vi "4309 multi test with switch.vi"() -> ()   [LabVIEW 2019]
uses:
  Chart_Graph_Mean_Range_StdDev.ctl
  <vilib>/Analysis/baseanly.llb/Mean (DBL).vi
  <vilib>/Analysis/NI_AALBase.lvlib
panel:
  in  "DMM 7.5 Digits All 4 Channels":dbl[][](array[numeric])=[[3.4835981189908805, 3.4835973578772146, 3.4835977893402292, 3.483597533766503, 3.4835975009361055, 3.4835974259988975, 3.4835978392404665, 3.483597710153336, 3.483597530409142, 3.483597982965577, 3.4835974835927273, 3.4835975661067864, 3.4835978929675346, 3.483597859704548, 3.483597570043803, 3.48359758877419, 3.483597718635417, 3.4835974386993853, 3.4835979909144443, 3.483597546796911, 3.483597791629489, 3.4835976928422, 3.4835977006392365, 3.4835976984527726, 3.4835973562416775, 3.483597995505588, 3.483597815535534, 3.4835978300326116, 3.483597985892642, 3.483597413809255, 3.483597723962119, 3.4835979022635915, 3.4835977166666647, 3.483597588468151, 3.483598009044623, 3.4835974566412133, 3.4835975839370192, 3.4835975376641026, 3.483597439503911, 3.483597317956866, 3.4835972485909776, 3.4835976458862903, 3.4835976825108617, 3.48359823081158, 3.4835976718930137, 3.4835976585808193, 3.4835978362135966, 3.483597507818025, 3.483597799164003, 3.483597349716458, 3.4835975948182454, 3.4835981329699433, 3.4835979467910407, 3.4835974912342884, 3.4835974532960456, 3.483597903200004, 3.483597374049583, 3.483597334623242, 3.483597710860957, 3.483597692009984, 3.4835976586327315, 3.4835977598936534, 3.4835979763023603, 3.4835975896116587, 3.4835978971434263, 3.4835976281822316, 3.4835982271082013, 3.4835976949272403, 3.4835974320575938, 3.483597408013519, 3.4835976534048685, 3.48359766337321, 3.483597430968089, 3.4835978228589006, 3.4835977691488273, 3.4835979109499484, 3.483597518460395, 3.483597806961959, 3.483597578691926, 3.4835975527599476, 3.483597860450459, 3.4835974511972227, 3.4835973978219275, 3.4835975280386107, 3.4835970961662297, 3.4835979186960975, 3.483597285920934, 3.483597386907896, 3.483597474535041, 3.4835973080741587, 3.4835975196582534, 3.4835974480673357, 3.4835976798422204, 3.483597547235268, 3.483597484346667, 3.483597539878841, 3.483597791092996, 3.483597598658644, 3.48359767066429, 3.4835976010356733, 3.4835977898228307, 3.483597544054286, 3.4835971331899516, 3.4835975044953993, 3.4835974626533996, 3.483597132727585, 3.4835975524889027, 3.4835979535117207, 3.4835972493429948, 3.483597640255253, 3.4835974086907697, 3.4835973506672318, 3.483597580088908, 3.483597239500539, 3.483597486011177, 3.4835975002194246, 3.483597090891085, 3.483597714859873, 3.4835976666442754, 3.4835972680152745, 3.4835977448807194, 3.483597350763673, 3.4835973529914943, 3.4835976118884404, 3.4835975154265597, 3.483597695000821, 3.4835974558961684, 3.483597790103636], [3.4850700897521563, 3.485070233425622, 3.4850703496943347, 3.4850708481529473, 3.485070572181595, 3.485070105960937, 3.485070465485683, 3.4850704480083396, 3.48507056459965, 3.4850708183835595, 3.4850708166846527, 3.485070796405387, 3.4850707761851427, 3.485070608667662, 3.4850707882696508, 3.4850707241151975, 3.4850706596362566, 3.48507073021978, 3.485070567481813, 3.4850707162760663, 3.485070893790592, 3.4850704393547267, 3.485070651192876, 3.485070267833332, 3.4850708914554103, 3.4850705970227684, 3.4850705496821712, 3.485070893808849, 3.485070908236491, 3.4850704723673553, 3.4850706194869305, 3.4850704541132527, 3.4850707021341325, 3.4850710097049173, 3.4850709609995607, 3.4850706992583946, 3.4850710502732944, 3.4850708242361663, 3.485071009568022, 3.4850706205187802, 3.4850704634402474, 3.4850708131553314, 3.485070283346761, 3.485070802639425, 3.4850707294320875, 3.4850710718142284, 3.48507067385808, 3.4850708139996227, 3.4850706485313316, 3.485071205234073, 3.4850708802082133, 3.485070539592214, 3.4850703284695643, 3.485070644610402, 3.4850706377352365, 3.485070724333666, 3.485070706865352, 3.485071039978291, 3.4850708932740937, 3.4850703374231804, 3.4850706519379795, 3.4850704993977777, 3.4850704497575355, 3.4850705472916865, 3.4850708830277983, 3.4850702392811503, 3.48507065435932, 3.4850707605356352, 3.4850706390730855, 3.4850704744759575, 3.4850708749760537, 3.4850704959682712, 3.48507057686368, 3.485070482100544, 3.485070110520969, 3.4850708314094643, 3.4850704513493116, 3.485070655338042, 3.4850698942787095, 3.485070641499467, 3.485070060001174, 3.485070454200556, 3.485070688596838, 3.4850706243046936, 3.485070579152903, 3.485069883099495, 3.485070062034084, 3.485070525913557, 3.485070210088132, 3.485070026034661, 3.4850702456185907, 3.485070243940185, 3.4850697001719446, 3.4850702521018917, 3.4850700772887624, 3.4850700859590287, 3.485070371774776, 3.4850700961734526, 3.485070172855618, 3.485069905757029, 3.4850703159307965, 3.4850698537426226, 3.485070462070553, 3.4850699512833727, 3.4850698464028094, 3.4850699259717026, 3.4850701371431896, 3.4850702401475635, 3.485070006300969, 3.485070088453557, 3.4850701595221656, 3.485070253223072, 3.4850696208469243, 3.4850698353777982, 3.48506973491397, 3.4850699043293396, 3.485069909154778, 3.485069945468628, 3.4850700162729797, 3.4850700637961176, 3.4850698568711835, 3.485069683841688, 3.485069930522382, 3.48506970179727, 3.485070116146578, 3.485070421850128, 3.485070158963441, 3.4850698427039397], [3.481571899555477, 3.4815720996809536, 3.481572168540679, 3.481572401004205, 3.4815723090577384, 3.481571988546094, 3.4815728274152624, 3.4815728062014335, 3.481572501577856, 3.481572607429995, 3.481572610595567, 3.4815725639158046, 3.4815731629523547, 3.48157245445838, 3.481572678822192, 3.481572529789867, 3.4815725819006804, 3.481572967069484, 3.4815731074475686, 3.481572693006066, 3.4815728208347263, 3.481572524099559, 3.481573131123811, 3.4815725324422293, 3.4815725721654815, 3.4815727955137086, 3.4815732409351097, 3.48157252834275, 3.481572511998337, 3.4815730302590793, 3.481572830362119, 3.4815731395241, 3.48157304282813, 3.481573010928663, 3.4815726753855367, 3.481573126747513, 3.4815728716190883, 3.481572781318836, 3.481572732683734, 3.4815727357820037, 3.481572704616765, 3.481572784355119, 3.4815728763523865, 3.4815728056849347, 3.481572474565925, 3.4815728651620326, 3.481572960730617, 3.4815730411537085, 3.4815726474348017, 3.4815728656925575, 3.4815728037625746, 3.4815725683714147, 3.4815727765135653, 3.481572602782018, 3.4815725196736356, 3.4815723014267093, 3.481572220656706, 3.481572534362172, 3.4815728413086053, 3.481572371815714, 3.481572564065832, 3.4815724851708483, 3.4815726220738314, 3.481572401586816, 3.481572213900522, 3.481572531080011, 3.4815726736061214, 3.481572174946321, 3.4815728025844557, 3.481572249370352, 3.4815721671205733, 3.481572565457693, 3.481572360373885, 3.4815726824797832, 3.481572841781139, 3.481572643049169, 3.4815721595516465, 3.4815723952810407, 3.481572162387346, 3.4815727239032985, 3.4815723917459103, 3.4815720794809555, 3.4815722693538627, 3.4815725743888026, 3.4815720485747352, 3.481572470689445, 3.4815725915569478, 3.4815727324723182, 3.4815724521032285, 3.4815727954319797, 3.4815721995573847, 3.4815721839029323, 3.4815721980816043, 3.4815721160737434, 3.481572277861212, 3.4815721507038226, 3.481572288856155, 3.481572226063303, 3.4815719656002706, 3.481572592875911, 3.481572194406493, 3.481572412416302, 3.481572084967407, 3.4815721696802724, 3.4815720226137596, 3.48157205650772, 3.48157190538414, 3.481572045063342, 3.481572018317761, 3.481572185489624, 3.481572154901699, 3.481571926660422, 3.4815718999626237, 3.4815721280737373, 3.481572224094029, 3.481572353081591, 3.481572261017972, 3.481571975995548, 3.481572128201471, 3.481572180067718, 3.4815715655143373, 3.4815718214629943, 3.4815715789142585, 3.4815719255662994, 3.4815718246399183, 3.481571977351035, 3.481571843104722, 3.4815719523213], [3.484305724115568, 3.4843058305875227, 3.4843062901111512, 3.484305936231965, 3.4843057288438772, 3.4843064559020687, 3.4843063293991383, 3.4843062952127486, 3.4843066955825175, 3.484306829330163, 3.4843061981418333, 3.4843063620415697, 3.484306236532934, 3.4843064437456763, 3.4843061743985606, 3.484306186782022, 3.484306270580653, 3.484306740665737, 3.4843061208250283, 3.484305965882024, 3.484306590076414, 3.4843059649148156, 3.4843062673844587, 3.4843060655731373, 3.484306302924423, 3.484306432337808, 3.484306632080742, 3.484306009373001, 3.484306543172826, 3.484306382441485, 3.4843062427876945, 3.4843061764316796, 3.48430660308128, 3.4843062004511594, 3.4843060610943404, 3.4843068333436076, 3.484306621812408, 3.484306649840404, 3.484306285295565, 3.4843059813072683, 3.484306553789793, 3.4843062824735846, 3.484306430756184, 3.4843068757434295, 3.484306442887929, 3.4843065762633945, 3.484305988738697, 3.4843066243270724, 3.484306445500346, 3.484306832441937, 3.4843060150056067, 3.4843063781220796, 3.4843066789757673, 3.4843064150739504, 3.4843061381565823, 3.484305675942912, 3.4843062793645334, 3.4843063841371547, 3.484306272484438, 3.4843062706304226, 3.484306376440192, 3.484305708893772, 3.484306251000281, 3.484306233665289, 3.4843063068999873, 3.4843062524955, 3.4843063590903363, 3.484305999586689, 3.4843062500567994, 3.4843060777149777, 3.484305966811333, 3.4843060316739654, 3.4843057546627394, 3.484306023228924, 3.4843061239924005, 3.4843060196427316, 3.4843055330739823, 3.4843056881987136, 3.484305713110319, 3.484306038013802, 3.484305910294656, 3.4843055487391927, 3.484305955637334, 3.4843058755725593, 3.4843058736827315, 3.4843058395981483, 3.4843057942888587, 3.4843056863141157, 3.484305964223715, 3.4843061658501737, 3.4843061897594634, 3.484305738279498, 3.484305518799016, 3.484305825857164, 3.484306035291972, 3.484306102538148, 3.484305819322618, 3.4843057482448683, 3.4843055381532038, 3.484305561533999, 3.48430561697876, 3.484305709331289, 3.484305709513193, 3.4843057764415675, 3.484305845716869, 3.4843058548617227, 3.4843058558332802, 3.4843060036480638, 3.484306017456, 3.4843051117756003, 3.4843054695551543, 3.484305914306639, 3.4843058242771217, 3.4843058614305953, 3.4843052097363807, 3.4843056026459474, 3.484305395133235, 3.4843055297155088, 3.484305541519446, 3.4843059349268186, 3.4843053694848685, 3.4843057348549347, 3.484305160045847, 3.484304944580094, 3.4843056614719075, 3.4843052011624254, 3.4843052966632158, 3.484305352531343]]
  in  "Take New DMM 7.5 Digit Measurements":bool
  out "error values of channels":dbl[][](array[numeric])=[[3.916877821419362e-05, 3.708869139362747e-06, 3.813682889530767e-05, 5.939885534989031e-06], [3.635893304743121e-05, -1.4762659956701896e-06, 3.541455057165521e-05, 6.165901756727266e-06], [3.8312583618971274e-05, 5.44234072030747e-07, 3.851021763967566e-05, 6.687408843131237e-06], [3.683071982907293e-05, 6.149038647151883e-07, 3.84443079650687e-05, 7.168960555414827e-06], [3.3856852708513685e-05, -2.440297388606183e-06, 3.5546966388633194e-05, 6.810853058869526e-06], [3.645943377117433e-05, 4.1571643194515673e-07, 3.861609064648164e-05, 7.510668457832992e-06], [3.376470219373928e-05, -2.523192756953563e-06, 3.560124494406125e-05, 7.423303348019772e-06], [3.310682505075491e-05, -1.8358768398840652e-06, 3.552758119029775e-05, 7.75010252906938e-06], [3.651997278319996e-05, 1.7017873870095457e-06, 3.969301297601646e-05, 8.367025434719011e-06], [3.8678501685485145e-05, 2.61423281289197e-06, 4.1762457464233904e-05, 1.1427786008599838e-05], [4.814853281098763e-05, 1.5347319277658755e-05, 4.9363542874658606e-05, 1.8916138766034152e-05], [5.463157506069294e-05, 2.148276930480364e-05, 5.719963653616489e-05, 3.198721146668859e-05]] format="%#_6p"
  out "Results Output":T1={"ch3 range"=1.4045208578838952e-05, "ch3 std dev"=3.830360581374409e-06, "ch3 mean"=3.484274052845448, "Histogram Graph ch3"={"X Values"=[3.484267646031002, 3.48426905055186, 3.4842704550727177, 3.4842718595935755, 3.4842732641144334, 3.4842746686352917, 3.4842760731561495, 3.4842774776770074, 3.484278882197865, 3.484280286718723], "Histogram: h(x)"=[2, 0, 1, 3, 2, 2, 1, 4, 0, 1]}, "ch2 range"=1.962617132944544e-05, "ch2 std dev"=5.564596788564025e-06, "ch2 mean"=3.4815152534979, "Histogram Graph ch2"={"X Values"=[3.4815041041457744, 3.481506066762907, 3.4815080293800404, 3.4815099919971733, 3.481511954614306, 3.4815139172314393, 3.481515879848572, 3.481517842465705, 3.481519805082838, 3.481521767699971], "Histogram: h(x)"=[2, 0, 0, 0, 3, 2, 2, 3, 1, 3]}, "ch1 range"=2.4894850890078146e-05, "ch1 std dev"=6.014144758608103e-06, "ch1 mean"=3.4850489507785483, "Histogram Graph ch1"={"X Values"=[3.4850381297721658, 3.4850406192572545, 3.4850431087423437, 3.485045598227433, 3.4850480877125216, 3.485050577197611, 3.4850530666826995, 3.4850555561677887, 3.485058045652878, 3.4850605351379667], "Histogram: h(x)"=[1, 1, 1, 3, 2, 4, 2, 1, 0, 1]}, "ch0 range"=2.9063497193337895e-05, "ch0 std dev"=7.35669530855736e-06, "ch0 mean"=3.4835429826473154, "Histogram Graph ch0"={"X Values"=[3.4835249461372704, 3.48352785248699, 3.483530758836709, 3.4835336651864286, 3.4835365715361477, 3.4835394778858673, 3.4835423842355864, 3.483545290585306, 3.483548196935025, 3.4835511032847446], "Histogram: h(x)"=[1, 0, 0, 2, 0, 2, 2, 3, 3, 3]}, "Waveform Chart ch1"=[3.485041350644882, 3.485053674025459, 3.485044470850417, 3.485051679765652, 3.485053893489457, 3.4850617798805112, 3.485044590124329, 3.4850435691396435, 3.4850485738729864, 3.485036885029621, 3.4850517417880864, 3.485044852526935, 3.4850504917974896, 3.4850485452472473, 3.485056627247517, 3.485050487026533], "Waveform Chart ch2"=[3.481503122837208, 3.4815117453734565, 3.481516626864648, 3.4815116069929637, 3.4815160351687457, 3.4815128237869555, 3.4815044398377637, 3.4815223290953163, 3.4815171040387627, 3.4815184592132473, 3.481520377453188, 3.4815227490085374, 3.4815136445264323, 3.481513673156879, 3.4815177577672993, 3.481521560844992], "Waveform Chart ch0"=[3.483545103302057, 3.483545418224207, 3.483538337247383, 3.483552556459604, 3.4835440249322716, 3.4835346774702782, 3.483523492962411, 3.4835479996315266, 3.4835430610796307, 3.4835471789253174, 3.4835508768748045, 3.4835475033905627, 3.483534453207535, 3.4835396637376506, 3.4835414148956656, 3.4835519600161384], "Waveform Chart ch3"=[3.4842715141883103, 3.4842764376445787, 3.4842719006223777, 3.4842773011577415, 3.484280988979152, 3.4842750302612457, 3.484271981725824, 3.4842737182937324, 3.4842669771661097, 3.484270526634582, 3.4842772200542953, 3.484277797320001, 3.4842735083789305, 3.4842749825533366, 3.484266943770573, 3.484278016776385]} {"ch3 range" format="%#_6p"; "ch3 std dev" format="%#.3p"; "ch3 mean" format="%#.6p"; "ch2 range" format="%#_6p"; "ch2 std dev" format="%#.3p"; "ch2 mean" format="%#.6p"; "ch1 range" format="%#_6p"; "ch1 std dev" format="%#.3p"; "ch1 mean" format="%#.6p"; "ch0 range" format="%#_6p"; "ch0 std dev" format="%#.3p"; "ch0 mean" format="%#.6p"}
  out "4309 Standard Deviation vs Aperture Time":T2(graph)={"Standard Deviation (Ohm)"=[0.0001, 0.0002, 0.001, 0.002, 0.005, 0.01, 0.016666666666666666, 0.03333333333333333, 0.05, 0.06666666666666667, 0.08333333333333333, 0.1], "Aperture Time (s)"=[6.685420033582732e-06, 4.157272478199315e-06, 2.0206962414231736e-06, 1.7721930677441643e-06, 1.3715901810211512e-06, 8.907703730682679e-07, 5.458658438864537e-07, 5.390458563910762e-07, 4.294169592032905e-07, 4.682861804544929e-07, 4.88865258212175e-07, 5.691708591765721e-07]}
  out "Aperture Time (s)":dbl[](array[numeric])=[0.0001, 0.0002, 0.001, 0.002, 0.005, 0.01, 0.016666666666666666, 0.03333333333333333, 0.05, 0.06666666666666667, 0.08333333333333333, 0.1] format="%#_6p"
  out "Sample Rates (Hz)":dbl[](array[numeric])=[10000.0, 5000.0, 1000.0, 500.0, 200.0, 100.0, 60.0, 30.0, 20.0, 15.0, 12.0, 10.0] format="%#_6p"
  out "Std Dev (V)":dbl[](array[numeric])=[6.685420033582732e-06, 4.157272478199315e-06, 2.0206962414231736e-06, 1.7721930677441643e-06, 1.3715901810211512e-06, 8.907703730682679e-07, 5.458658438864537e-07, 5.390458563910762e-07, 4.294169592032905e-07, 4.682861804544929e-07, 4.88865258212175e-07, 5.691708591765721e-07] format="%#_6p"
  out "Range (V)":dbl[](array[numeric])=[2.697917404170802e-05, 1.523478858311833e-05, 6.77997672804409e-06, 6.631974495574511e-06, 4.914311322989917e-06, 3.161019406450194e-06, 1.956195919472492e-06, 1.992032487851958e-06, 1.767743138758604e-06, 1.579287696840126e-06, 1.5983576289180235e-06, 1.9418800938364456e-06] format="%#_6p"
  out "Elapsed Time (ms)":u32[](array[numeric])=[118, 170, 258, 238, 398, 707, 1177, 2209, 3243, 4311, 5376, 6507]
  out "4309 mean values of channels":dbl[][](array[numeric])=[[3.483558445444162, 3.4850667246787137, 3.4815343163055408, 3.48430010017138], [3.4835612552893287, 3.4850719098138487, 3.4815370385838644, 3.484299874155158], [3.483559301638757, 3.485069889313781, 3.4815339429167964, 3.4842993526480717], [3.483560783502547, 3.4850698186439883, 3.481534008826471, 3.4842988710963594], [3.4835637573696676, 3.4850728738452417, 3.4815369061680475, 3.484299229203856], [3.483561154788605, 3.485070017831421, 3.4815338370437896, 3.484298529388457], [3.4835638495201824, 3.48507295674061, 3.481536851889492, 3.484298616753567], [3.4835645073973254, 3.485072269424693, 3.481536925553246, 3.4842982899543857], [3.483561094249593, 3.485068731760466, 3.48153276012146, 3.48429767303148], [3.4835589357206906, 3.48506781931504, 3.481530690676972, 3.484294612270906], [3.483549465689565, 3.4850550862285754, 3.4815230895915614, 3.4842871239181488], [3.4835429826473154, 3.4850489507785483, 3.4815152534979, 3.484274052845448]]
  out "error out":errorcluster
  in  "error in":errorcluster
  in  "Rates":dbl[](array[numeric])=[10.0, 12.0, 15.0, 20.0, 30.0, 60.0, 100.0, 200.0, 500.0, 1000.0, 5000.0, 10000.0] format="%#_6p"
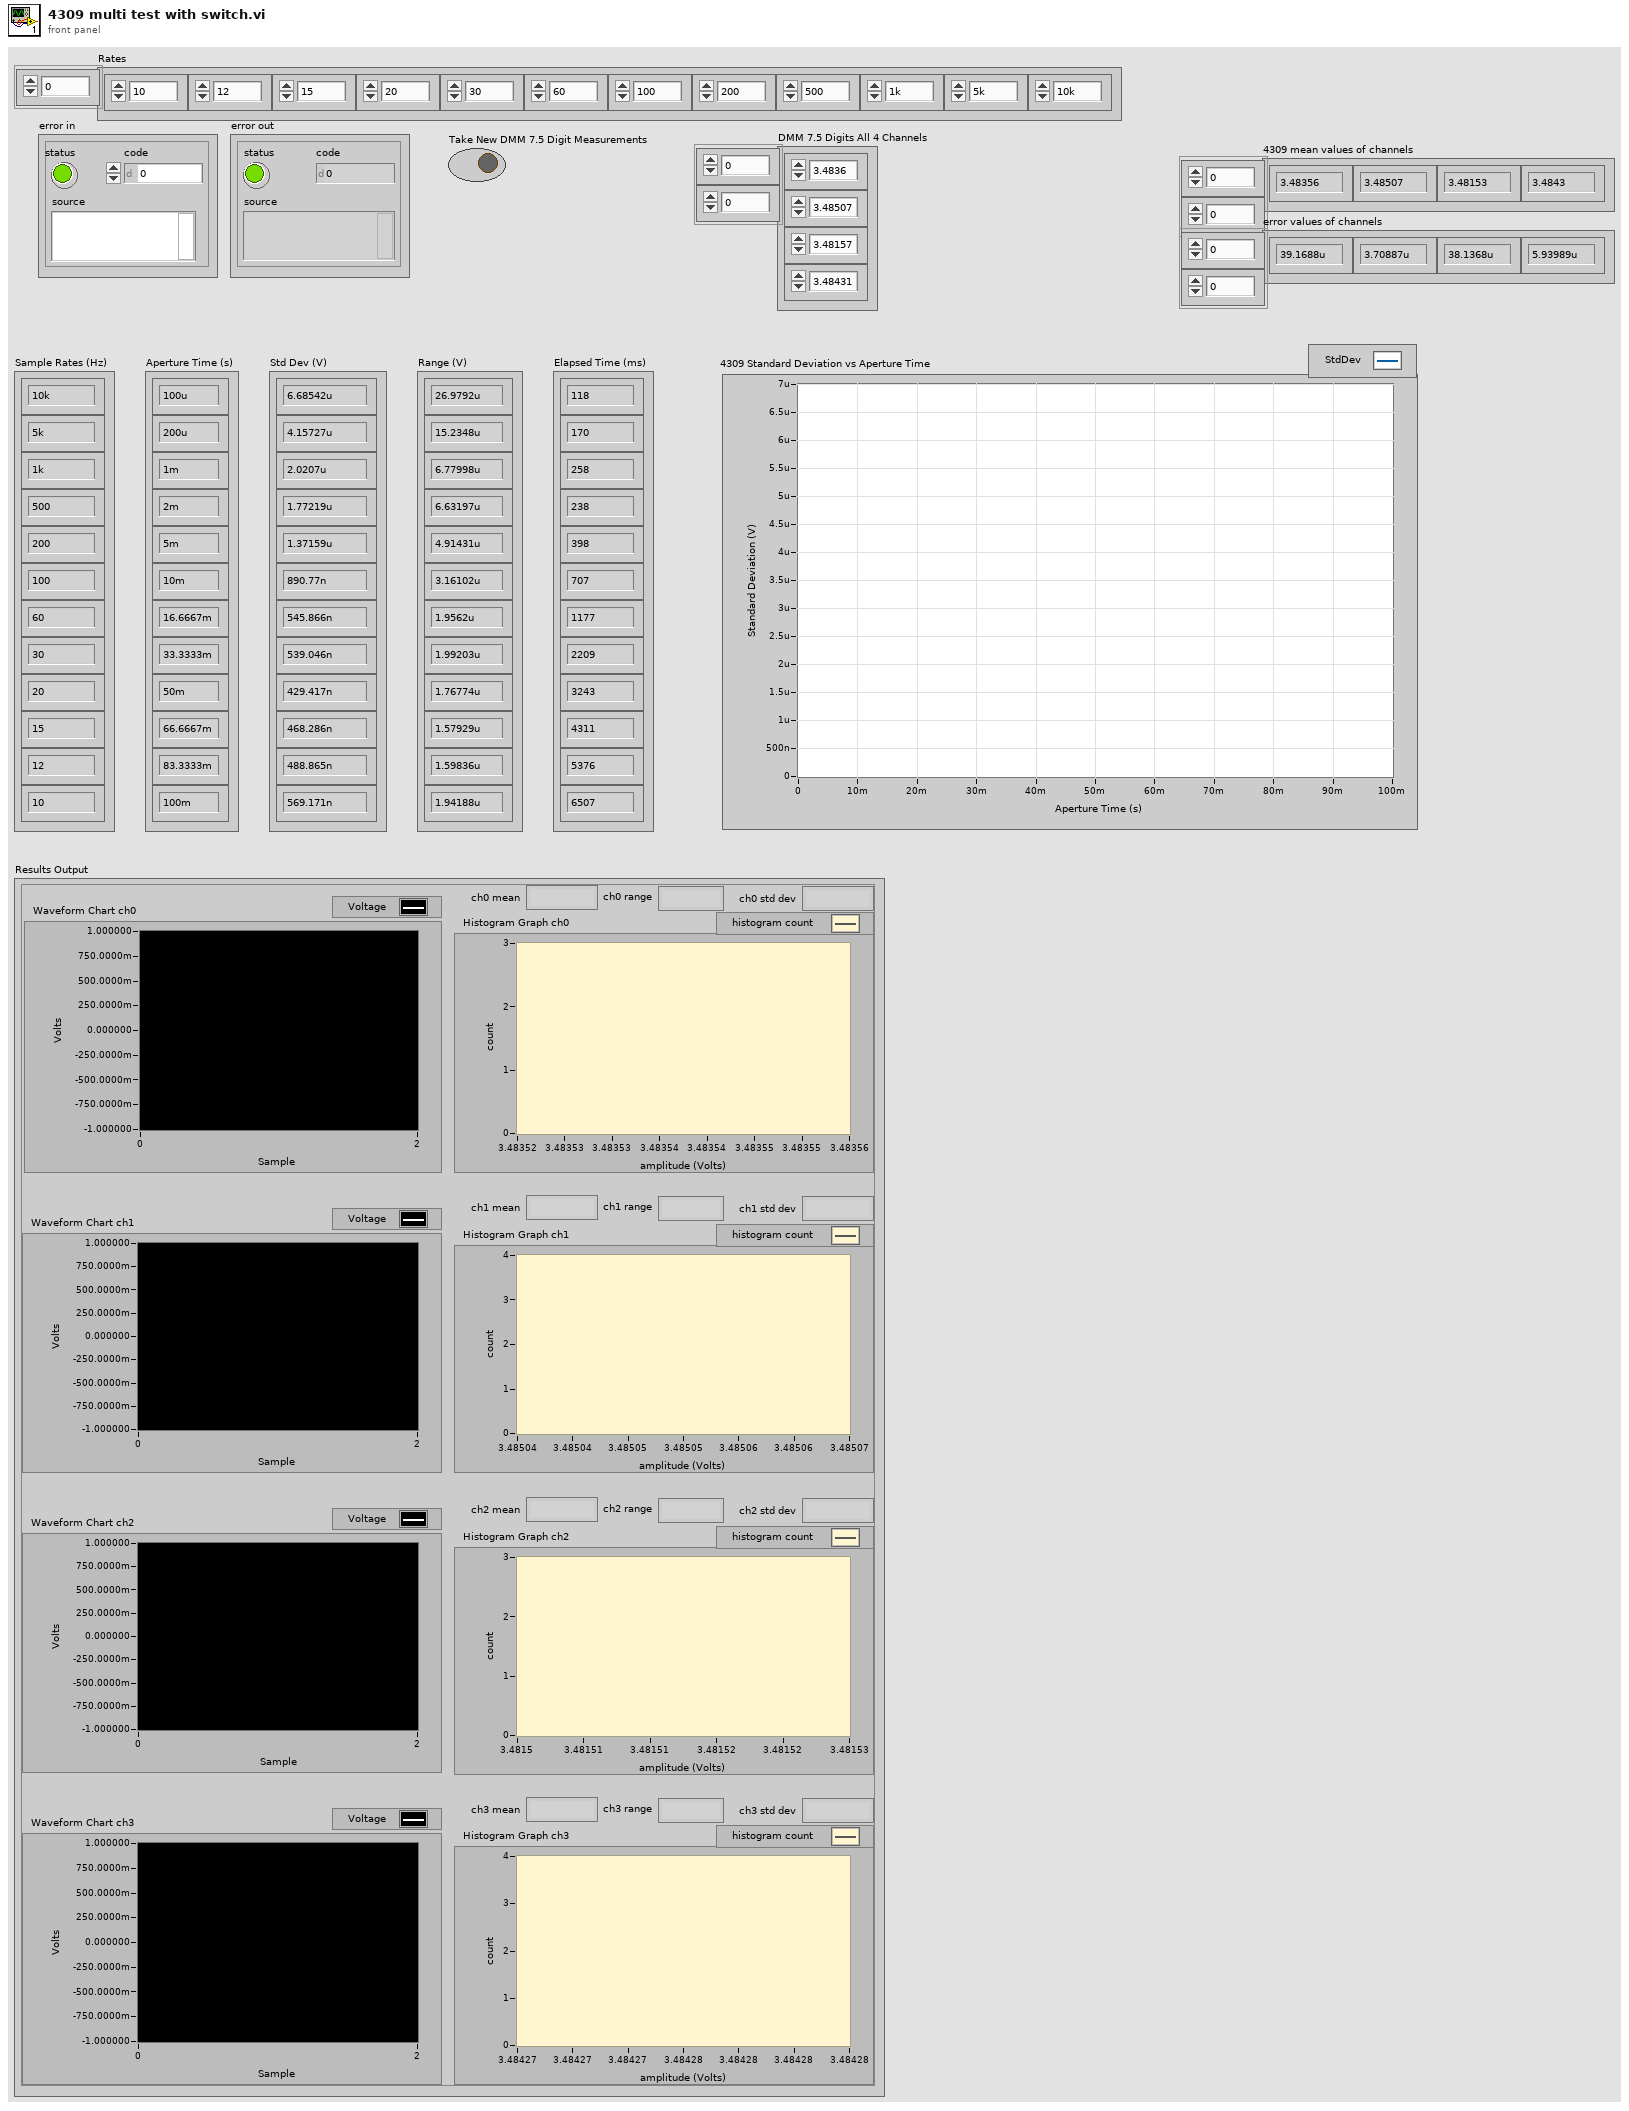
[diagram p1: front panel]
types:
  T1 = typedef "Chart_Graph_Mean_Range_StdDev.ctl" = cluster{"ch3 range":dbl, "ch3 std dev":dbl, "ch3 mean":dbl, "Histogram Graph ch3":cluster{"X Values":dbl[], "Histogram: h(x)":i32[]}, "ch2 range":dbl, "ch2 std dev":dbl, "ch2 mean":dbl, "Histogram Graph ch2":cluster{"X Values":dbl[], "Histogram: h(x)":i32[]}, "ch1 range":dbl, "ch1 std dev":dbl, "ch1 mean":dbl, "Histogram Graph ch1":cluster{"X Values":dbl[], "Histogram: h(x)":i32[]}, "ch0 range":dbl, "ch0 std dev":dbl, "ch0 mean":dbl, "Histogram Graph ch0":cluster{"X Values":dbl[], "Histogram: h(x)":i32[]}, "Waveform Chart ch1":dbl[], "Waveform Chart ch2":dbl[], "Waveform Chart ch0":dbl[], "Waveform Chart ch3":dbl[]}
  T2 = cluster{"Standard Deviation (Ohm)":dbl[], "Aperture Time (s)":dbl[]}
  T3 = typedef "OCVResults.ctl" = cluster{"V ch0 Array":dbl[], "V ch1 Array":dbl[], "V ch2 Array":dbl[], "V ch3 Array":dbl[], "V ch4 Array":dbl[], "Elapsed Time (ms)":u32, "DMM Fault Array":bool[]}
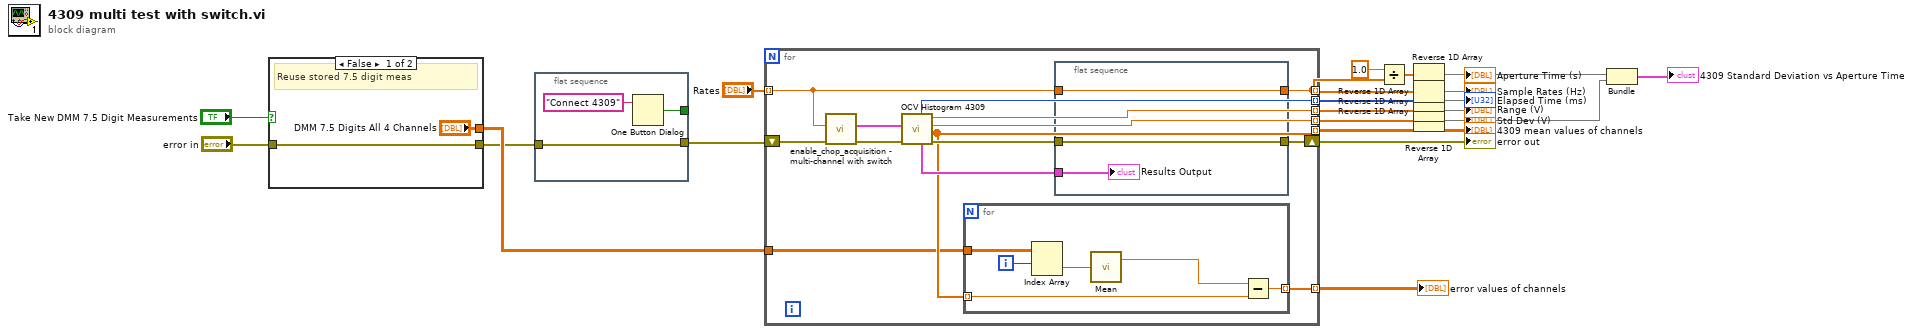
[diagram p0: block diagram]
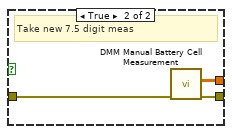
[diagram p2: hidden frame]
diagram:
  n1 = case shown="False" "Take New DMM 7.5 Digit Measurements" {
    tunnel: "error in" -> [w23 w26]
    tunnel: ["DMM 7.5 Digits All 4 Channels" w25] -> w10
    tunnel: [w23 w24] -> w9
    frame False {
      # "Reuse stored 7.5 digit meas"
    }
    frame True {
      # "Take new 7.5 digit meas"
      n2 = call "DMM Manual Battery Cell Measurement.vi"("error in"=w26) -> ("error out"=w24:errorcluster, "Measurements (Volts) All"=w25:dbl[][])  [unwired: 9 in]
    }
  }
  n3 = flat-sequence {
    tunnel: w9 -> [w28]
    tunnel: [w28] -> w8
    tunnel: [w27] -> _
    frame #0 {
      n4 = One Button Dialog(message="Connect 4309") -> (true=w27:bool)  [unwired: 1 in]
    }
  }
  n5 = for {
    shift-right: [w36] -> w21
    shift-left: w8 -> [w33]
    tunnel: [w41] -> w17 mode=indexing
    tunnel: [w40] -> w16 mode=indexing
    tunnel: [w39] -> w13 mode=indexing
    tunnel: [w32] -> w20 mode=indexing
    tunnel: [w34] -> w18 mode=indexing
    tunnel: "Rates" -> [w35] mode=indexing
    tunnel: [w31] -> w12 mode=indexing
    tunnel: w10 -> [w30]
    n6 = call "enable_chop_acquisition - multi-channel with switch.vi"("error in"=w33, "rate (Hz)"=w35) -> ("error out"=w43:errorcluster, "Results"=w42:T3)  [unwired: 8 in]
    n7 = call "OCV Histogram 4309.vi"("Error In"=w43, "Results Input"=w42) -> ("Error Out"=w37:errorcluster, "mean values of channels"=w32:dbl[], "std dev"=w39:dbl, "range"=w40:dbl, "Results Output"=w38:T1, "Elapsed Time (ms)"=w41:u32)  [unwired: 4 in]
    n8 = for {
      tunnel: w32 -> [w49] mode=indexing
      tunnel: [w48] -> w31 mode=indexing
      tunnel: w30 -> [w47]
      i -> [w46]
      n9 = Index Array(array=w47, index (row)=w46) -> (element=w45:dbl[])  [unwired: 1 in]
      n10 = call-poly <vilib>:"Mean.vi"("X"=w45) -> ("mean"=w44:dbl)  [unwired: 1 out]
      n11 = Subtract(x=w44, y=w49) -> (x-y=w48:dbl)
    }
    n12 = flat-sequence {
      tunnel: w38 -> [w52]
      tunnel: w37 -> [w51]
      tunnel: [w51] -> w36
      tunnel: w35 -> [w50]
      tunnel: [w50] -> w34
      frame #0 {
        "Results Output" <- w52
      }
    }
  }
  "error out" <- w21
  "4309 mean values of channels" <- w20
  "error values of channels" <- w12
  n13 = Divide(x=1.0, y=w18) -> (x/y=w14:dbl[])
  n14 = Reverse 1D Array(array=w14) -> (reversed array=w1:dbl[])
  "Aperture Time (s)" <- w1
  n15 = Reverse 1D Array(array=w18) -> (reversed array=→"Sample Rates (Hz)":dbl[])
  n16 = Reverse 1D Array(array=w17) -> (reversed array=→"Elapsed Time (ms)":u32[])
  n17 = Reverse 1D Array(array=w16) -> (reversed array=→"Range (V)":dbl[])
  n18 = Reverse 1D Array(array=w13) -> (reversed array=w2:dbl[])
  "Std Dev (V)" <- w2
  n19 = Bundle(w1, w2) -> (→"4309 Standard Deviation vs Aperture Time":cluster{dbl[], dbl[]})  [unwired: 1 in]
